vi "Instrument Type ID.vi"() -> (1 "instrument type id":string="Keysight34401A_DMM")   [LabVIEW 2025, in "Keysight 34461A DMM Instrument.lvlib"]
uses:
  Keysight 34461A DMM Instrument.lvlib
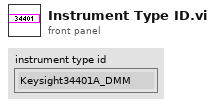
[diagram p1: front panel]
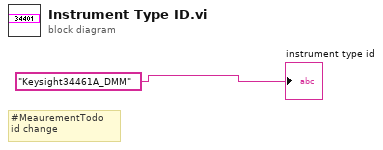
[diagram p0: block diagram]
diagram:
  # "#MeaurementTodo\nid change"
  "instrument type id" <- "Keysight34461A_DMM" ("instrument_type_id")
